vi "Draw_ColDet.vi"(5 "Background Alpha":dbl=0.5, 7 "Background Color":u32(colorbox)=13750737, 8 "error in":errorcluster) -> (0 "error out":errorcluster)   [LabVIEW 2011]
doc: "This VI will draw the current scene. Objects displayed in blue have no collision, object dark red have a AABB collision and objects in red have a mesh collision."
uses:
  Enflo_Collision_Detection.dll
  <vilib>/picture/3D Picture Control/NI_3D Picture Control.lvlib
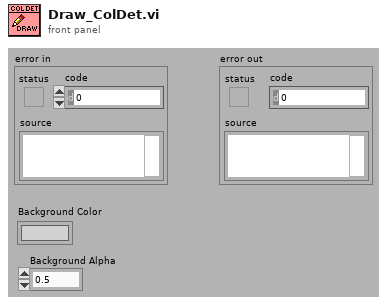
[diagram p1: front panel]
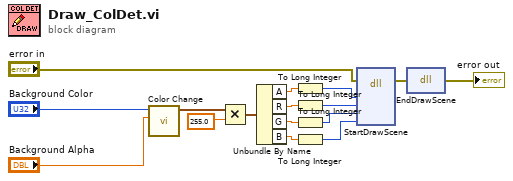
[diagram p0: block diagram]
diagram:
  n1 = call <vilib>:"Color Change.vi"("Alpha"="Background Alpha", "Color"="Background Color") -> ("RGBA"=w11:cluster{"R":sgl, "G":sgl, "B":sgl, "A":sgl})  [unwired: 9 in]
  n2 = Multiply(x=w11, y=sgl 255.0 ("R")) -> (x*y=w9:cluster{"R":sgl, "G":sgl, "B":sgl, "A":sgl})
  n3 = Unbundle By Name(w9) -> ("A"=w5:sgl, "R"=w6:sgl, "G"=w7:sgl, "B"=w8:sgl)
  n4 = To Long Integer(number=w5) -> (32bit integer=w4:i32)
  n5 = To Long Integer(number=w6) -> (32bit integer=w3:i32)
  n6 = To Long Integer(number=w7) -> (32bit integer=w2:i32)
  n7 = To Long Integer(number=w8) -> (32bit integer=w1:i32)
  n8 = dll-call lib="C:/Enflo_Software_SVN/EnFloSW/Anemometry/Anemometry Sub Vis/Collision_Detection/Enflo_Collision_Detection.dll" fn="StartDrawScene"(error in="error in", "A"=w4, "R"=w3, "G"=w2, "B"=w1) -> (error out=w15:errorcluster)  [unwired: 7 in, 1 out]
  n9 = dll-call lib="C:/Enflo_Software_SVN/EnFloSW/Anemometry/Anemometry Sub Vis/Collision_Detection/Enflo_Collision_Detection.dll" fn="EndDrawScene"(error in=w15) -> (error out=→"error out":errorcluster)  [unwired: 3 in, 1 out]
